vi "Sphere-in-Box test (object-oriented).vi"(1 "Box":T2, 2 "Sphere":T1) -> (0 "Sphere is inside box":bool)   [LabVIEW 2014]
uses:
  Typedefs/TreeNodeBox.ctl
  Typedefs/Quad.ctl
  Typedefs/Quadplane enum.ctl
  Typedefs/Sphere.ctl
panel:
  # "PN 13/03/2015"
  # "Vertices"
  # "Edges"
  # "Unit normal"
  # "Plane ident."
  # "Vertices"
  # "Edges"
  # "Unit normal"
  # "Plane ident."
  # "Vertices"
  # "Edges"
  # "Unit normal"
  # "Plane ident."
  # "Vertices"
  # "Edges"
  # "Unit normal"
  # "Plane ident."
  # "Vertices"
  # "Edges"
  # "Unit normal"
  # "Plane ident."
  # "Vertices"
  # "Edges"
  # "Unit normal"
  # "Plane ident."
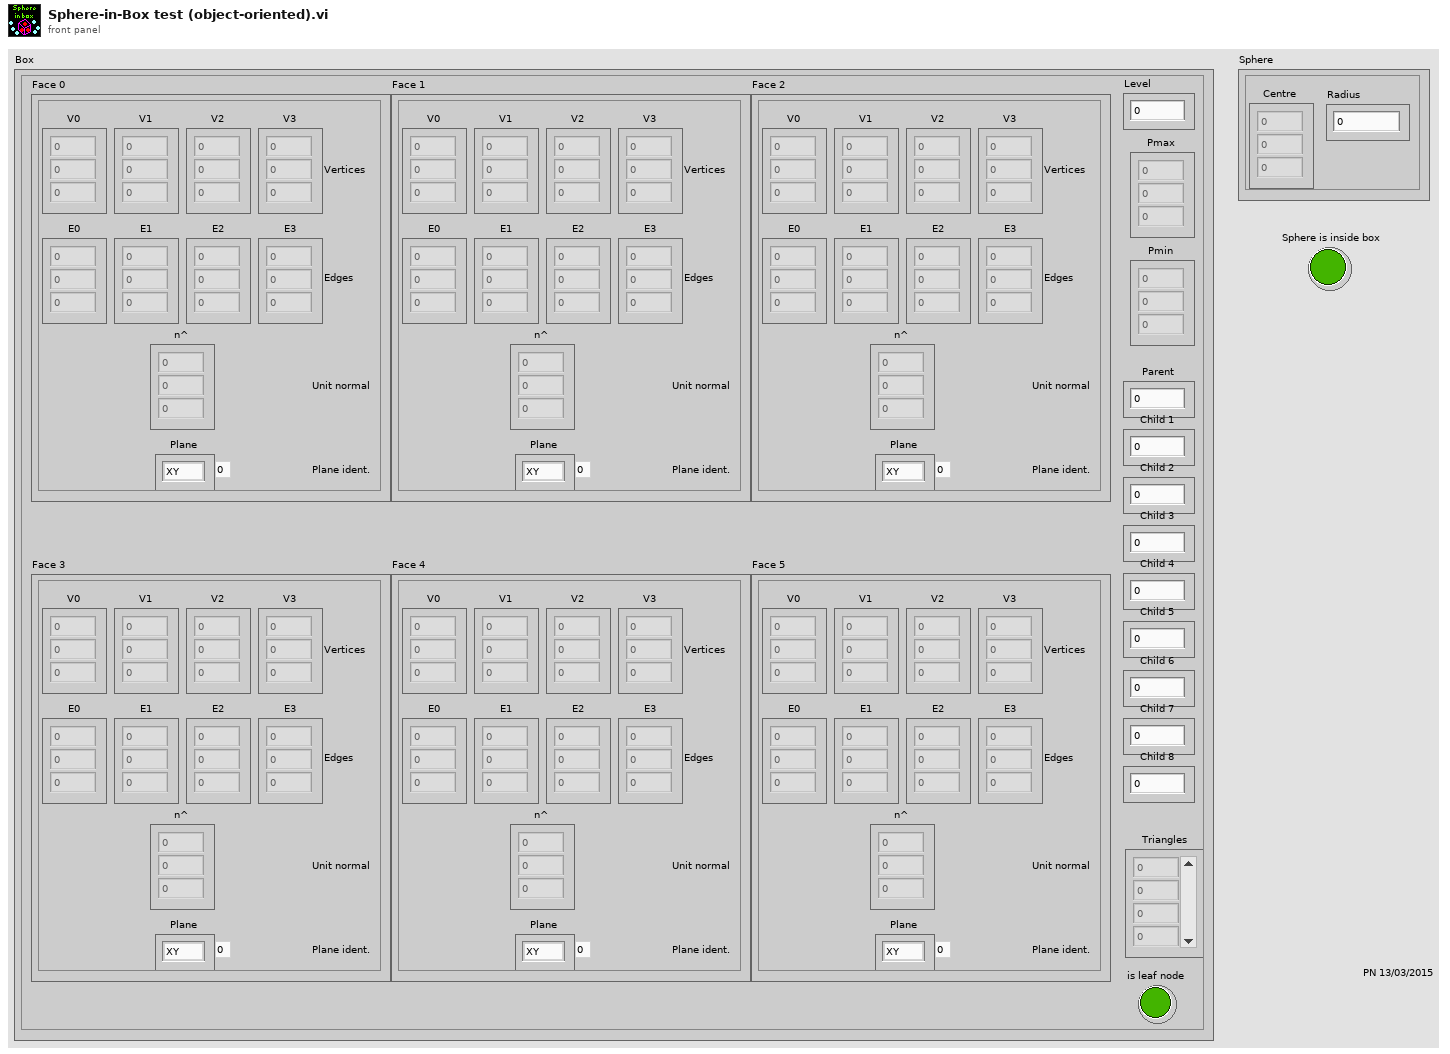
[diagram p1: front panel]
types:
  T1 = typedef "Sphere.ctl" = cluster{"Centre":sgl[], "Radius":sgl}
  T2 = typedef "TreeNodeBox.ctl" = cluster{"Face 0":T3, "Face 1":T3, "Face 2":T3, "Face 3":T3, "Face 4":T3, "Face 5":T3, "Level":i32, "Pmax":sgl[], "Pmin":sgl[], "Parent":i32, "Child 1":i32, "Child 2":i32, "Child 3":i32, "Child 4":i32, "Child 5":i32, "Child 6":i32, "Child 7":i32, "Child 8":i32, "Triangles":i32[], "is leaf node":bool}
  T3 = typedef "Quad.ctl" = cluster{"V0":sgl[], "V1":sgl[], "V2":sgl[], "V3":sgl[], "E0":sgl[], "E1":sgl[], "E2":sgl[], "E3":sgl[], "n^":sgl[], "Plane":T4}
  T4 = typedef "Quadplane enum.ctl" = enum8{"XY", "XZ", "YZ", "-XY", "-XZ", "-YZ"}
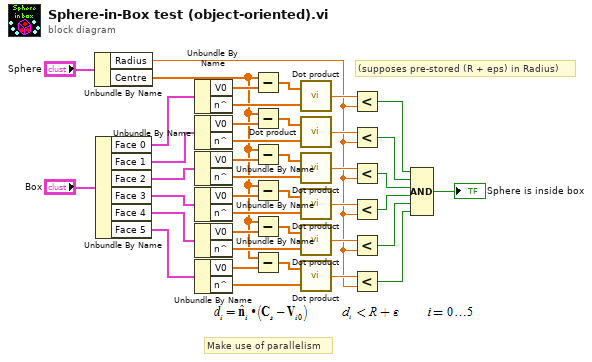
[diagram p0: block diagram]
diagram:
  # "(supposes pre-stored (R + eps) in Radius)"
  # "Make use of parallelism"
  n1 = Unbundle By Name("Sphere") -> ("Radius"=w1:sgl, "Centre"=w2:sgl[])
  n2 = Unbundle By Name("Box") -> ("Face 0"=w40:T3, "Face 1"=w39:T3, "Face 2"=w38:T3, "Face 3"=w37:T3, "Face 4"=w36:T3, "Face 5"=w35:T3)
  n3 = Unbundle By Name(w40) -> ("V0"=w34:sgl[], "n^"=w28:sgl[])
  n4 = Unbundle By Name(w39) -> ("V0"=w33:sgl[], "n^"=w21:sgl[])
  n5 = Unbundle By Name(w38) -> ("V0"=w32:sgl[], "n^"=w20:sgl[])
  n6 = Unbundle By Name(w37) -> ("V0"=w31:sgl[], "n^"=w19:sgl[])
  n7 = Unbundle By Name(w36) -> ("V0"=w30:sgl[], "n^"=w18:sgl[])
  n8 = Unbundle By Name(w35) -> ("V0"=w29:sgl[], "n^"=w17:sgl[])
  n9 = Subtract(x=w2, y=w34) -> (x-y=w27:sgl[])
  n10 = Subtract(x=w2, y=w33) -> (x-y=w26:sgl[])
  n11 = Subtract(x=w2, y=w32) -> (x-y=w25:sgl[])
  n12 = Subtract(x=w2, y=w31) -> (x-y=w24:sgl[])
  n13 = Subtract(x=w2, y=w30) -> (x-y=w23:sgl[])
  n14 = Subtract(x=w2, y=w29) -> (x-y=w22:sgl[])
  n15 = call "Dot product.vi"("B"=w28, "A"=w27) -> ("A . B"=w16:sgl)
  n16 = call "Dot product.vi"("B"=w21, "A"=w26) -> ("A . B"=w15:sgl)
  n17 = call "Dot product.vi"("B"=w20, "A"=w25) -> ("A . B"=w14:sgl)
  n18 = call "Dot product.vi"("B"=w19, "A"=w24) -> ("A . B"=w13:sgl)
  n19 = call "Dot product.vi"("B"=w18, "A"=w23) -> ("A . B"=w12:sgl)
  n20 = call "Dot product.vi"("B"=w17, "A"=w22) -> ("A . B"=w11:sgl)
  n21 = Less?(x=w16, y=w1) -> (x < y?=w10:bool)
  n22 = Less?(x=w15, y=w1) -> (x < y?=w9:bool)
  n23 = Less?(x=w14, y=w1) -> (x < y?=w8:bool)
  n24 = Less?(x=w13, y=w1) -> (x < y?=w7:bool)
  n25 = Less?(x=w12, y=w1) -> (x < y?=w6:bool)
  n26 = Less?(x=w11, y=w1) -> (x < y?=w5:bool)
  n27 = Compound Arithmetic op=AND(w10, w9, w8, w7, w6, w5) -> (→"Sphere is inside box":bool)
